vi "S-Curve.vi"() -> ()   [LabVIEW 2020]
uses:
  <vilib>/Analysis/1siggen.llb/Ramp Pattern by Samples.vi
  <vilib>/Analysis/NI_AALBase.lvlib
panel:
  in  "Asymmetry \nFactor":dbl
  out "Waveform Graph":waveform(dbl)(graph)
  out "Charge (mC)":dbl
  in  "Steepness\nFactor":dbl
  in  "Recharge\nAmplitude (mA)":dbl
  in  "Recharge\nCurve Time (s)":dbl
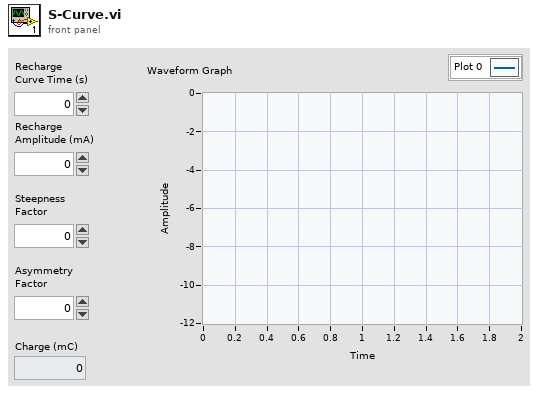
[diagram p1: front panel]
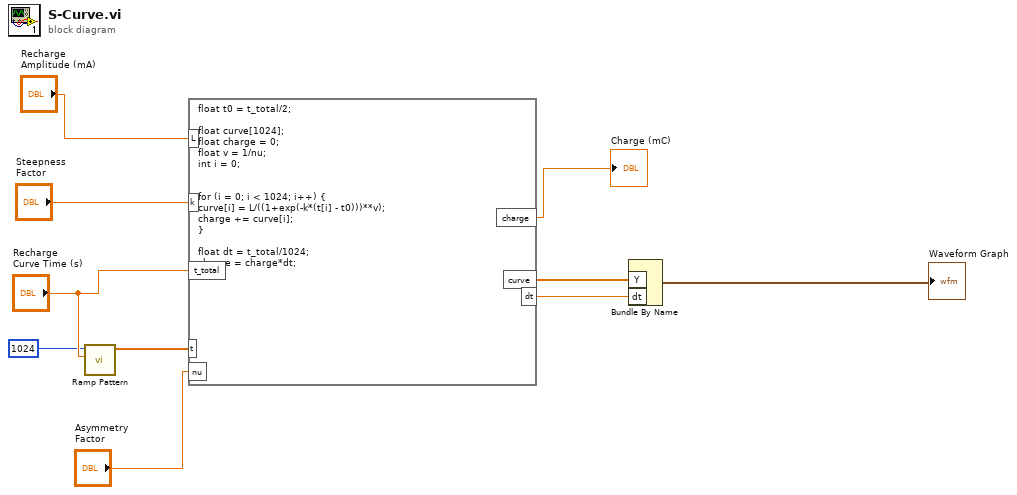
[diagram p0: block diagram]
diagram:
  n1 = call-poly <vilib>:"Ramp Pattern.vi"("end"="Recharge\nCurve Time (s)", "samples"=1024) -> ("Ramp Pattern"=w5:dbl[])  [unwired: 8 in, 1 out]
  n2 = formula code="float t0 = t_total/2;\n\nfloat curve[1024];\nfloat charge = 0;\nfloat v = 1/nu;\nint i = 0;\n\n\nfor (i = 0; i < 1024; i++) {\ncurve[i] = L/((1+exp(-k*(t[i] - t0)))**v);\ncharge += curve[i];\n}\n\nfloat dt = t_total/1024;\ncharge = charge*dt;"("L"="Recharge\nAmplitude (mA)", "k"="Steepness\nFactor", "t_total"="Recharge\nCurve Time (s)", "t"=w5, "nu"="Asymmetry \nFactor") -> ("charge"=→"Charge (mC)":dbl, "curve"=w4:dbl[], "dt"=w3:dbl)
  n3 = Bundle By Name("Y"=w4, "dt"=w3) -> (→"Waveform Graph":waveform(dbl))  [unwired: 1 in]
